vi "PH_uOPA_DelayController.Control Loop.vi"(0 "VI in":refnum<vi>, 2 "uOPA Peak":dbl, 5 "error in (no error)":errorcluster) -> (14 "VI out":refnum<vi>, 16 "Control Status":T1, 19 "error out":errorcluster)   [LabVIEW 2014, in "PH_uOPA_DelayController.lvlib"]
uses:
  PH_uOPA_DelayController.lvlib
  PH_uOPA_DelayController.Control Status.ctl
  PH_Basics/PH_Stepmotor_BaseClass/PH_Stepmotor_BaseClass.Axis Direction.ctl
  <vilib>/ptbypt/NI_PtbyPt.lvlib
  PH_Basics/PH_Common/PH_Common.lvlib
  PH_Basics/PH_AxisGUI_BaseClass/PH_AxisGUI_BaseClass.lvlib
  PH_Basics/PH_Stepmotor_BaseClass/PH_Stepmotor_BaseClass.lvlib
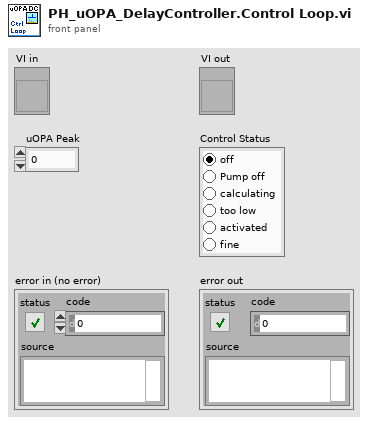
[diagram p1: front panel]
types:
  T1 = typedef "PH_uOPA_DelayController.lvlib/PH_uOPA_DelayController.Control Status.ctl" = enum32{"off", "Pump off", "calculating", "too low", "activated", "fine"}
  T2 = typedef "PH_Stepmotor_BaseClass.lvlib/PH_Stepmotor_BaseClass.Axis Direction.ctl" = enum16{"forward", "backward"}
  T3 = typedef "PH_uOPA_DelayController.lvlib/PH_uOPA_DelayController.i attribute.ctl" = cluster{"GUI Refs":cluster{"Current Pump Peak":refnum<vi>, "Current uOPA Peak":refnum<vi>, "Pump Peak":refnum<vi>, "uOPA Peak":refnum<vi>, "uOPA Target":refnum<vi>, "uOPA Limits [%]":refnum<vi>, "sample length":refnum<vi>, "Pump Target":refnum<vi>, "Pump Limit":refnum<vi>, "Pump running":refnum<vi>, "Feedback Control":refnum<vi>, "Control Status":refnum<vi>, "uOPA Mean":refnum<vi>, "Current uOPA Mean":refnum<vi>}, "uOPA Target":dbl, "uOPA Limits [%]":T4, "Sample Length":i32, "Initialize Mean":bool, "Pump Target":dbl, "Pump Limit [%]":dbl, "Feedback Control":bool, "Control Status":T1, "last Mean":dbl, "last direction":T2, "Axis Settings":T5, "Width while feedback":dbl}
  T4 = typedef "PH_uOPA_DelayController.lvlib/PH_uOPA_DelayController.Limit.ctl" = cluster{"low":dbl, "activate":dbl, "fine":dbl}
  T5 = typedef "PH_Stepmotor_BaseClass.lvlib/PH_Stepmotor_BaseClass.Axis Settings.ctl" = cluster{"Sign change":bool, "Width":dbl, "Calibration":dbl, "Unit":string, "Motor Type":T6, "Unit Width":string, "Unit CF":string}
  T6 = typedef "PH_Stepmotor_BaseClass.lvlib/PH_Stepmotor_BaseClass.Motor Type.ctl" = enum16{"Unspecific", "OWIS 49.120.2633", "OWIS 49.060.1033", "OWIS 43.040.2558", "Diamond Motion 2200 series", "OWIS 49.120.266B.MV6", "Calorimeter", "Linear Stage 1", "MICOS VT-80", "MICOS VT-80 S", "Standa Rotstage nt0.95A", "PUF RA 320.200", "PUF RA 800.200", "PUF RA 800.400", "PUF RA 400.50", "1324.nn.800.50", "1324.n9c.800.50", "1324.nn.320.200", "1324.nn.400.200", "1324.nn.800.200", "1324.nn.400.50", "1324.8c9c.800.50", "1324.8c9c.400.200"}
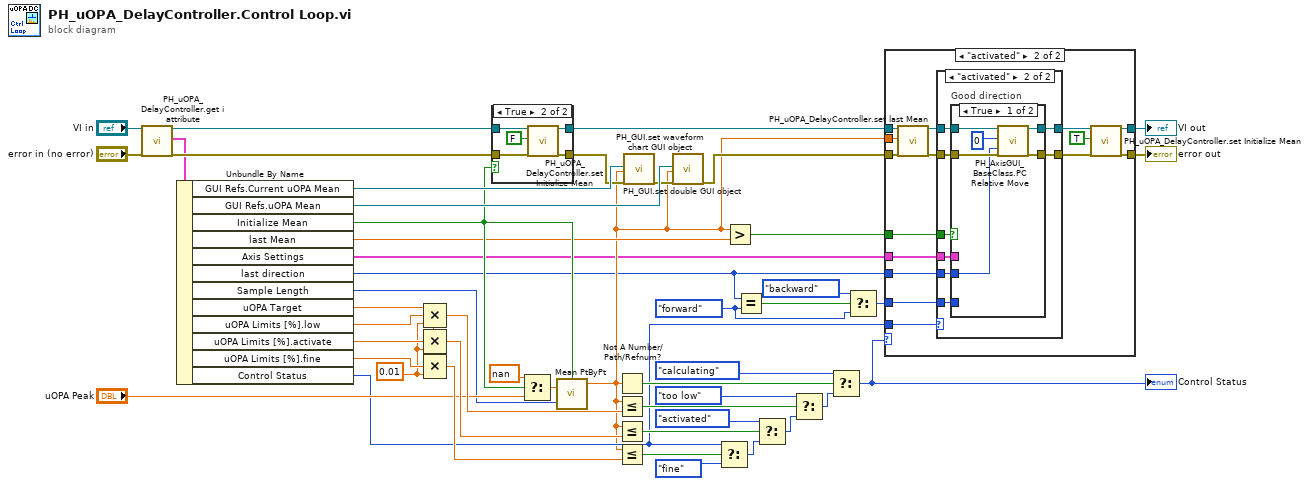
[diagram p0: block diagram]
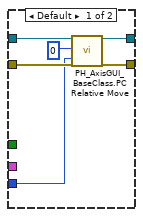
[diagram p3: hidden frame]
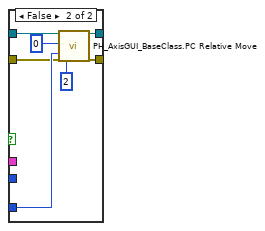
[diagram p4: hidden frame]
diagram:
  w6 = PH_Stepmotor_BaseClass.Axis_Direction."forward" ("last direction")
  w38 = 0.01 ("value")
  n1 = call "PH_uOPA_DelayController.get i attribute.vi"("i ref in"="VI in", "error in (no error)"="error in (no error)") -> ("i ref out"=w47:refnum<vi>, "i attribute"=w34:T3, "error out"=w48:errorcluster)  [unwired: 15 in]
  n2 = Unbundle By Name(w34) -> ("GUI Refs.Current uOPA Mean"=w37:refnum<vi>, "GUI Refs.uOPA Mean"=w36:refnum<vi>, "Initialize Mean"=w35:bool, "last Mean"=w9:dbl, "Axis Settings"=w1:T5, "last direction"=w2:T2, "Sample Length"=w10:i32, "uOPA Target"=w39:dbl, "uOPA Limits [%].low"=w13:dbl, "uOPA Limits [%].activate"=w40:dbl, "uOPA Limits [%].fine"=w41:dbl, "Control Status"=w11:T1)
  n3 = Compound Arithmetic op=MULTIPLY(w39, w13, w38) -> (w42:dbl)
  n4 = Compound Arithmetic op=MULTIPLY(w39, w40, w38) -> (w43:dbl)
  n5 = Compound Arithmetic op=MULTIPLY(w39, w41, w38) -> (w44:dbl)
  n6 = case shown="True" w35 {
    tunnel: w48 -> [w49 w55]
    tunnel: [w49 w51] -> w33
    tunnel: w47 -> [w50 w54]
    tunnel: [w50 w52] -> w14
    frame False {
    }
    frame True {
      n7 = call "PH_uOPA_DelayController.set Initialize Mean.vi"("VI in"=w54, "Initialize Mean? (True)"=FALSE, "error in (no error)"=w55) -> ("VI out"=w52:refnum<vi>, "error out"=w51:errorcluster)  [unwired: 15 in]
    }
  }
  n8 = Select(t=nan, s=w35, f="uOPA Peak") -> (s? t:f=w20:dbl)
  n9 = call <vilib>:"Mean PtByPt.vi"("x"=w20, "sample length"=w10, "initialize"=w35) -> ("mean"=w8:dbl)  [unwired: 1 in, 1 out]
  n10 = Not A Number/Path/Refnum?(number/path/refnum=w8) -> (NaN/Path/Refnum?=w21:bool)
  n11 = Less Or Equal?(x=w8, y=w42) -> (x <= y?=w23:bool)
  n12 = Less Or Equal?(x=w8, y=w43) -> (x <= y?=w26:bool)
  n13 = Less Or Equal?(x=w8, y=w44) -> (x <= y?=w28:bool)
  n14 = call "PH_GUI.set double GUI object.vi"("GUI object Ref"=w37, "value"=w8, "error in (no error)"=w33) -> ("error out"=w32:errorcluster)  [unwired: 16 in]
  n15 = call "PH_GUI.set waveform chart GUI object.vi"("WaveformChart in"=w36, "Double"=w8, "error in (no error)"=w32) -> ("error out"=w17:errorcluster)  [unwired: 16 in]
  n16 = Select(t=w11, s=w28, f=PH_uOPA_DelayController.Control_Status."fine" ("Control Status")) -> (s? t:f=w30:T1)
  n17 = Greater?(x=w8, y=w9) -> (0:w7:bool)
  n18 = Equal?(x=w2, y=w6) -> (x = y?=w5:bool)
  n19 = Select(t=PH_uOPA_DelayController.Control_Status."activated" ("Control Status"), s=w26, f=w30) -> (s? t:f=w27:T1)
  n20 = Select(t=PH_uOPA_DelayController.Control_Status."too low" ("Control Status"), s=w23, f=w27) -> (s? t:f=w25:T1)
  n21 = Select(t=PH_uOPA_DelayController.Control_Status."calculating" ("Control Status"), s=w21, f=w25) -> (s? t:f=w12:T1)
  "Control Status" <- w12
  n22 = Select(t=PH_Stepmotor_BaseClass.Axis_Direction."backward" ("last direction"), s=w5, f=w6) -> (s? t:f=w3:T2)
  n23 = case shown="\"activated\"" w12 {
    tunnel: w17 -> [w56 w72]
    tunnel: [w56 w60] -> w16
    tunnel: [w57 w62] -> w15
    tunnel: w14 -> [w57 w71]
    tunnel: w8 -> [_ w70]
    tunnel: w11 -> [_ w69]
    tunnel: w2 -> [_ w66]
    tunnel: w7 -> [_ w65]
    tunnel: w3 -> [_ w64]
    tunnel: w1 -> [_ w58]
    frame Default {
    }
    frame "activated" {
      n24 = call "PH_uOPA_DelayController.set last Mean.vi"("VI in"=w71, "Last Mean"=w70, "error in (no error)"=w72) -> ("VI out"=w68:refnum<vi>, "error out"=w67:errorcluster)  [unwired: 15 in]
      n25 = case shown="\"activated\"" w69 {
        tunnel: w68 -> [w77 w86]
        tunnel: [w76 w85] -> w61
        tunnel: w67 -> [w75 w84]
        tunnel: [w74 w83] -> w59
        tunnel: w66 -> [w73 w82]
        tunnel: w65 -> [_ w81]
        tunnel: w64 -> [_ w80]
        tunnel: w58 -> [_ w79]
        frame Default {
          n26 = call "PH_AxisGUI_BaseClass.PC Relative Move.vi"("i ref in"=w77, "Axis"=0, "direction"=w73, "error in"=w75) -> ("i ref out"=w76:refnum<vi>, "error out"=w74:errorcluster)  [unwired: 14 in]
        }
        frame "activated" {
          n27 = case "Good direction" shown="True" w81 {
            tunnel: w86 -> [w92 w96]
            tunnel: [w91 w95] -> w85
            tunnel: w84 -> [w90 w97]
            tunnel: [w89 w94] -> w83
            tunnel: w82 -> [w87 _]
            tunnel: w80 -> [_ w99]
            tunnel: w79 -> [_ _]
            frame True {
              n28 = call "PH_AxisGUI_BaseClass.PC Relative Move.vi"("i ref in"=w92, "Axis"=0, "direction"=w87, "error in"=w90) -> ("i ref out"=w91:refnum<vi>, "error out"=w89:errorcluster)  [unwired: 14 in]
            }
            frame False {
              n29 = call "PH_AxisGUI_BaseClass.PC Relative Move.vi"("i ref in"=w96, "Axis"=0 ("index"), "direction"=w99, "error in"=w97, "Multiple (1)"=2) -> ("i ref out"=w95:refnum<vi>, "error out"=w94:errorcluster)  [unwired: 13 in]
            }
          }
        }
      }
      n30 = call "PH_uOPA_DelayController.set Initialize Mean.vi"("VI in"=w61, "Initialize Mean? (True)"=TRUE, "error in (no error)"=w59) -> ("VI out"=w62:refnum<vi>, "error out"=w60:errorcluster)  [unwired: 15 in]
    }
  }
  "error out" <- w16
  "VI out" <- w15
